vi "ingest.csv.vi"(8 "error in":errorcluster, 9 "Path":path, 10 "dataset_rid":string, 11 "TabularIngestStaging in":refnum<class "TabularIngestStaging.lvclass">) -> (0 "error out":errorcluster, 3 "TabularIngestStaging out":refnum<class "TabularIngestStaging.lvclass">)   [LabVIEW 2020, in "TabularIngestStaging.lvclass"]
doc: "Ingests a CSV file from the given path into an existing dataset."
uses:
  TabularIngestStaging.lvclass
  TabularIngestStaging.lvclass/TabularIngestStaging.ctl
  client.lvlib
panel:
  out "out_job out":i32
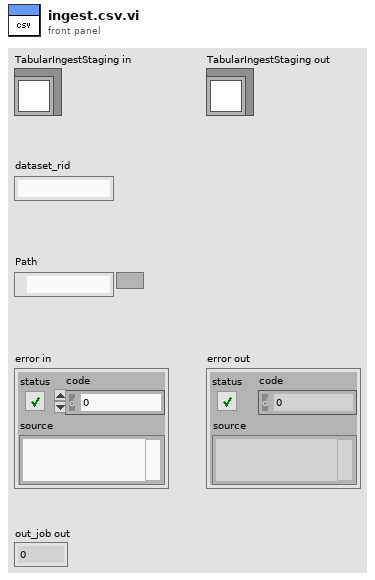
[diagram p1: front panel]
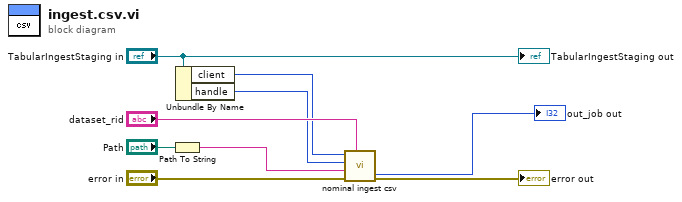
[diagram p0: block diagram]
diagram:
  n1 = Path To String(path="Path") -> (string=w2:string)
  n2 = Unbundle By Name("TabularIngestStaging in") -> ("client"=w4:i32, "handle"=w5:i32)
  n3 = call "nominal ingest csv.vi"("dataset_rid"="dataset_rid", "error in (no error)"="error in", "file_path"=w2, "staging"=w5, "client"=w4) -> ("error out"=→"error out":errorcluster, "out_job out"=→"out_job out":i32)  [unwired: 4 in, 1 out]
  "TabularIngestStaging out" <- "TabularIngestStaging in"
